vi "PlatMods to Rclick mods.vi"(11 "PlatMods":T2) -> (3 "Rclick mods":T1)   [LabVIEW 2021, in "RocketPlot.lvlib"]
uses:
  RocketPlot.lvlib
  TypeDefs/RightClickCache PlatMod.ctl
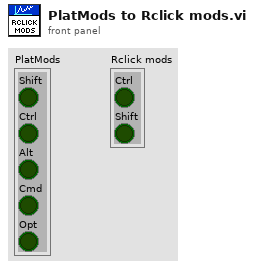
[diagram p1: front panel]
types:
  T1 = typedef "RocketPlot.lvlib/RightClickCache PlatMod.ctl" = cluster{"Ctrl":bool, "Shift":bool}
  T2 = cluster{"Shift":bool, "Ctrl":bool, "Alt":bool, "Cmd":bool, "Opt":bool}
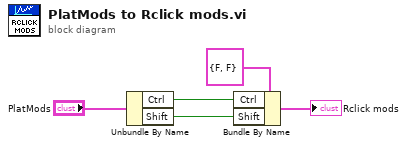
[diagram p0: block diagram]
diagram:
  n1 = Unbundle By Name("PlatMods") -> ("Ctrl"=w3:bool, "Shift"=w1:bool)
  n2 = Bundle By Name(cluster=T1 {"Ctrl"=FALSE, "Shift"=FALSE} ("RightClickCache.Mod"), "Ctrl"=w3, "Shift"=w1) -> (→"Rclick mods":T1)
